vi "Other Output Item Init.vi"(7 "Project In":refnum<class "Project.lvclass">, 8 "error in (no error)":errorcluster, 9 "Other UI Elements":T1, 10 "Output":T2, 11 "VI in":refnum<vi>) -> (0 "error out":errorcluster)   [LabVIEW 2015, in "OutputUI.lvclass"]
uses:
  OutputUI.lvclass
  Step/STEP_OUTPUT.ctl
  Step/OUTPUT_DATA_TYPE.ctl
  OUTPUT_CHECK_TYPE.ctl
  Step/OUTPUT_VALUE_TYPE.ctl
  Project.lvclass
  Step.lvclass
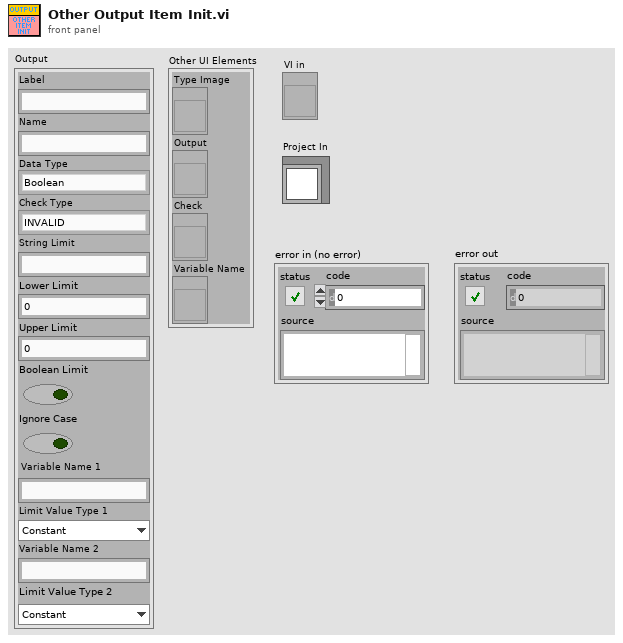
[diagram p1: front panel]
types:
  T1 = cluster{"Type Image":refnum<vi>, "Output":refnum<vi>, "Check":refnum<vi>, "Variable Name":refnum<vi>}
  T2 = typedef "Step.lvclass/STEP_OUTPUT.ctl" = cluster{"Label":string, "Name":string, "Data Type":T3, "Check Type":T4, "String Limit":string, "Lower Limit":dbl, "Upper Limit":dbl, "Boolean Limit":bool, "Ignore Case":bool, "Variable Name 1":string, "Limit Value Type 1":T5, "Variable Name 2":string, "Limit Value Type 2":T5}
  T3 = typedef "Step.lvclass/OUTPUT_DATA_TYPE.ctl" = enum16{"Boolean", "String", "Numeric", "Other"}
  T4 = typedef "Step.lvclass/OUTPUT_CHECK_TYPE.ctl" = enum16{"INVALID", "DO_NOT_CHECK", "RECORD", "VARIABLE", "EQUAL", "NOT_EQUAL", "STR_CONTAINS", "STR_START_WITH", "STR_END_WITH", "STR_REGEX_MATCH", "NUM_GT", "NUM_LT", "NUM_GE", "NUM_LE", "NUM_RANGE", "NUM_RANGE_BDY"}
  T5 = typedef "Step.lvclass/OUTPUT_VALUE_TYPE.ctl" = enum16{"Constant", "Variable"}
  T6 = cluster{"Type Image":refnum<vi>, "Output":refnum<vi>, "Check":refnum<vi>}
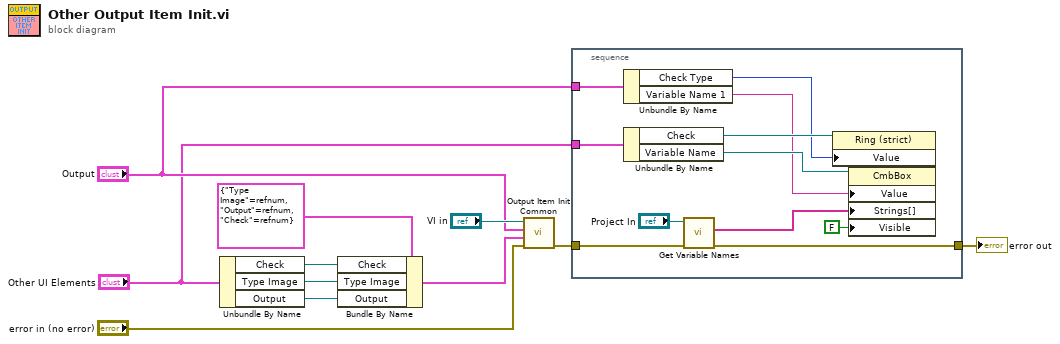
[diagram p0: block diagram]
diagram:
  n1 = Unbundle By Name("Other UI Elements") -> ("Check"=w9:refnum<vi>, "Type Image"=w8:refnum<vi>, "Output"=w7:refnum<vi>)
  n2 = Bundle By Name(cluster=T6 {"Type Image"=refnum, "Output"=refnum, "Check"=refnum} ("UI Elements"), "Check"=w9, "Type Image"=w8, "Output"=w7) -> (w5:T6)
  n3 = call "Output Item Init Common.vi"("error in (no error)"="error in (no error)", "UI Elements"=w5, "Output"="Output", "VI in"="VI in") -> ("error out"=w2:errorcluster)  [unwired: 7 in]
  n4 = stacked-sequence {
    tunnel: "Output" -> [w22]
    tunnel: "Other UI Elements" -> [w21]
    tunnel: w2 -> [w15]
    tunnel: [w14] -> w11
    frame #0 {
      n5 = Unbundle By Name(w22) -> ("Check Type"=w19:T4, "Variable Name 1"=w17:string)
      n6 = Unbundle By Name(w21) -> ("Check"=w20:refnum<vi>, "Variable Name"=w18:refnum<vi>)
      n7 = call "Get Variable Names.vi"("error in (no error)"=w15, "Project in"="Project In") -> ("error out"=w14:errorcluster, "Variable Names"=w13:string[])  [unwired: 7 in, 1 out]
      n8 = property class="Ring (strict)"(reference=w20, "Value"=w19) -> ()  [unwired: 1 in, 2 out]
      n9 = property class="CmbBox"(reference=w18, "Value"=w17, "Strings[]"=w13, "Visible"=FALSE) -> ()  [unwired: 1 in, 2 out]
    }
  }
  "error out" <- w11
